vi "check if running.vi"(8 "error in (no error)":errorcluster, 11 "Stepper in":refnum<class "Stepper.lvclass">) -> (0 "error out":errorcluster, 2 "Running?":bool, 3 "Stepper out":refnum<class "Stepper.lvclass">)   [LabVIEW 2025, in "Motor.lvlib" / "Stepper.lvclass"]
uses:
  Stepper.lvclass
  Stepper.lvclass/Stepper.ctl
panel:
  out "Waveform Chart":u16(graph)
  out "register":u16 format="%.0b"
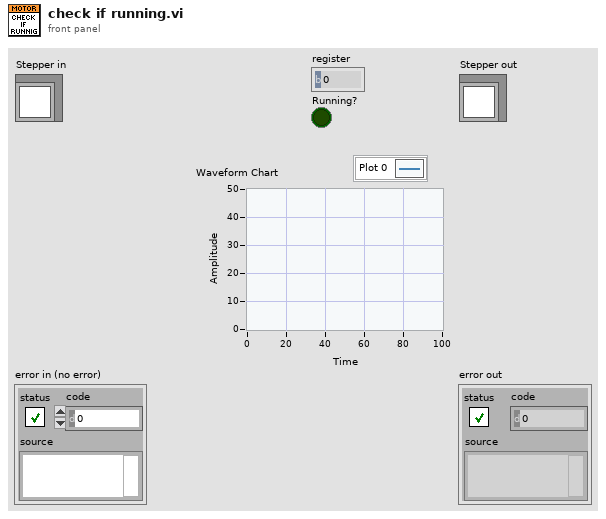
[diagram p1: front panel]
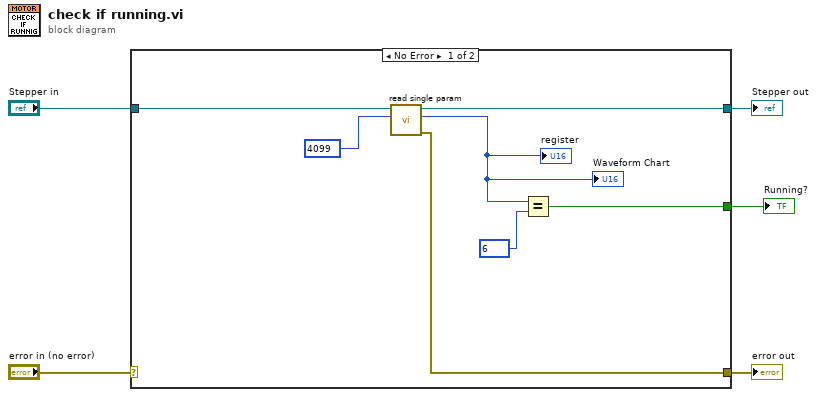
[diagram p0: block diagram]
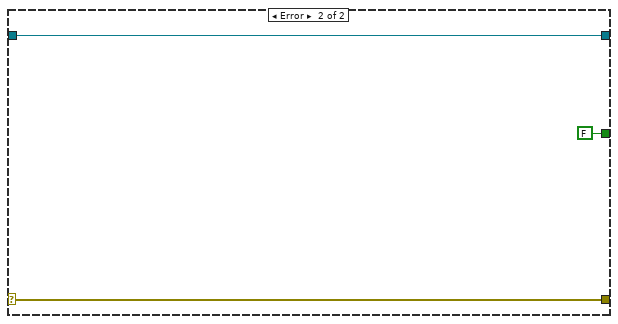
[diagram p2: hidden frame]
diagram:
  n1 = case shown="No Error" "error in (no error)" {
    selector: "error in (no error)" -> [_ w15]
    tunnel: [w9 w15] -> w4
    tunnel: [w11 w14] -> w2
    tunnel: "Stepper in" -> [w12 w14]
    tunnel: [w7 FALSE] -> w1
    frame No Error {
      n2 = call-dynamic "read single param.vi"("address"=u16 4099, "Stepper in"=w12) -> ("error out"=w9:errorcluster, "register"=w6:u16, "Stepper out"=w11:refnum<class "Stepper.lvclass">)  [unwired: 7 in]
      "register" <- w6
      "Waveform Chart" <- w6
      n3 = Equal?(x=w6, y=u16 6 ("address")) -> (x = y?=w7:bool)
    }
    frame Error {
    }
  }
  "error out" <- w4
  "Stepper out" <- w2
  "Running?" <- w1
